vi "TimedDoor_Create.vi"(0 "reference in":refnum<class "TimedDoor.lvclass">, 5 "error in (no error)":errorcluster) -> (14 "reference out":refnum<class "TimedDoor.lvclass">, 19 "error out":errorcluster)   [LabVIEW 2020, in "TimedDoor.lvclass"]
uses:
  TimedDoor.lvclass
  C:/Projects/DesignPatterns_Trunk/Timer/Door_class/Door.lvclass
  TimedDoor.lvclass/TimedDoor.ctl
  TimedDoor_ITimerTimeout_interface/TimedDoor_ITimerTimeout.lvclass
  C:/Projects/DesignPatterns_Trunk/Timer/ITimerTimeout_Interface/ITimerTimeout.lvclass
  Door_class/Door.lvclass
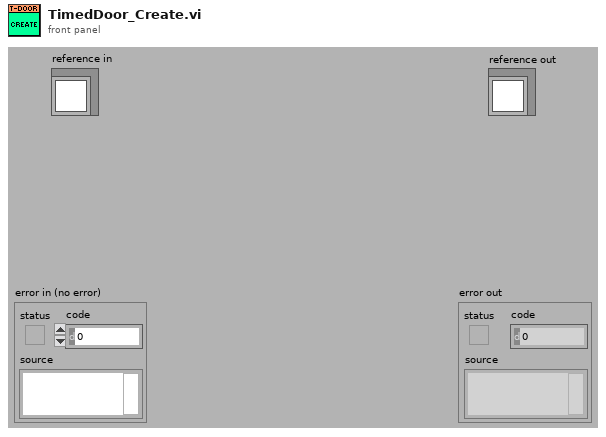
[diagram p1: front panel]
types:
  T1 = typedef "G4SubTemplate_Simple_6x8x6.lvclass/ObjectAttributes.ctl" = cluster{"Attribute1":dbl}
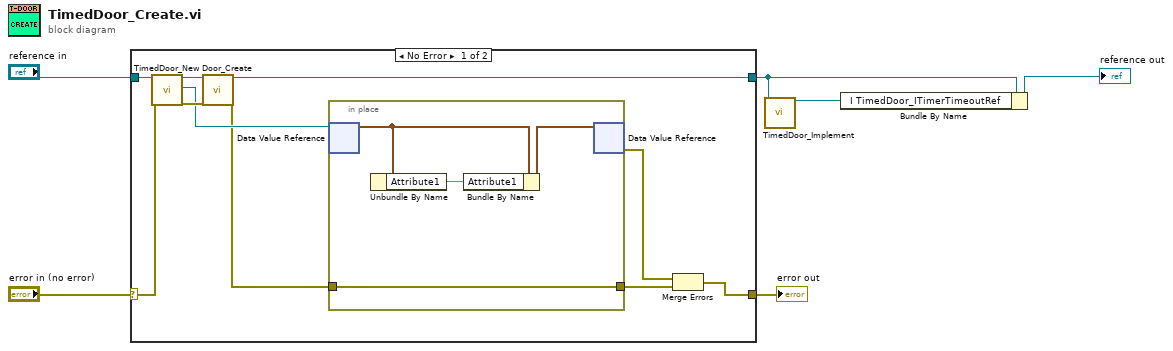
[diagram p0: block diagram]
diagram:
  n1 = case shown="No Error" "error in (no error)" {
    selector: "error in (no error)" -> [w15 w22]
    tunnel: [w13 w22] -> w5
    tunnel: "reference in" -> [w16 w21]
    tunnel: [w10 w21] -> w2
    frame No Error {
      n2 = call "TimedDoor_New.vi"("reference in"=w16, "error in (no error)"=w15) -> ("reference out"=w12:refnum<class "TimedDoor.lvclass">, "DVRRefOut"=w9:refnum<data-value>, "error out"=w11:errorcluster)  [unwired: 14 in, 1 out]
      n3 = call "Door_Create.vi"("reference in"=w12, "error in (no error)"=w11) -> ("reference out"=w10:refnum<class "TimedDoor.lvclass">, "error out"=w8:errorcluster)  [unwired: 16 in]
      n4 = in-place {
        in-place-border: w8 -> [w17]
        in-place-border: [w17] -> w7
        n5 = in-place-dvr #1(w9) -> (w19:T1)  [unwired: 1 out]
        n6 = Unbundle By Name(w19) -> ("Attribute1"=w18:dbl)
        n7 = Bundle By Name(cluster=w19, "Attribute1"=w18) -> (w20:T1)
        n8 = in-place-dvr #1(w20) -> (w14:errorcluster)  [unwired: 1 out]
      }
      n9 = Merge Errors(w14, w7) -> (w13:errorcluster)
    }
    frame Error {
    }
  }
  "error out" <- w5
  n10 = call "TimedDoor_Implement.vi"("ClassThatImplements"=w2) -> ("InterfaceHelpClass"=w1:refnum<class "TimedDoor_ITimerTimeout.lvclass">)  [unwired: 10 in]
  n11 = Bundle By Name(cluster=w2, "I TimedDoor_ITimerTimeoutRef"=w1) -> (→"reference out":refnum<class "TimedDoor.lvclass">)
